vi "gRPC_Wrapper_VISA_implement_v1.1.0.vi"() -> ()   [LabVIEW 2022 SP3]
uses:
  <vilib>/Instr/_visa.llb/VISA Open Access Mode.ctl
panel:
  out "Read in sec":dbl
  out "Write in sec":dbl
  out "Round Trip Time (ms)":dbl
  out "Read time":timestamp
  out "Write time":timestamp
  in  "Refresh":bool
  in  "VISA CLOSE":bool
  in  "VISA resource name":refnum<visa-resource-name>="test_LabVIEW"
  out "Waveform Graph":dbl[](graph)
  out "Waveform Chart":dbl(graph)
  out "Gain":string
  in  "Select Command":string(combo)
  out "Active":bool
  in  "Send":bool
  in  "Type Command":string
  in  "Query":bool
  out "Command":string
  out "Dot-Notation Address":string
  out "Computer Hostname":string
  out "Resource Manufacturer Name":string
  out "Resource Manufacturer Identification":u16
  out "Version of Specification":u32
  out "Resource Lock State":u32(ring) items=["Unlocked", "Exclusive", "Shared"]
  out "Resource Name":string
  out "Read return count":u32
  out "Write return count":u32
  out "Respose From Device":string
  # "Operations"
  # "Informations"
  # "Device Signal Parameters"
  # "Graph / Chart"
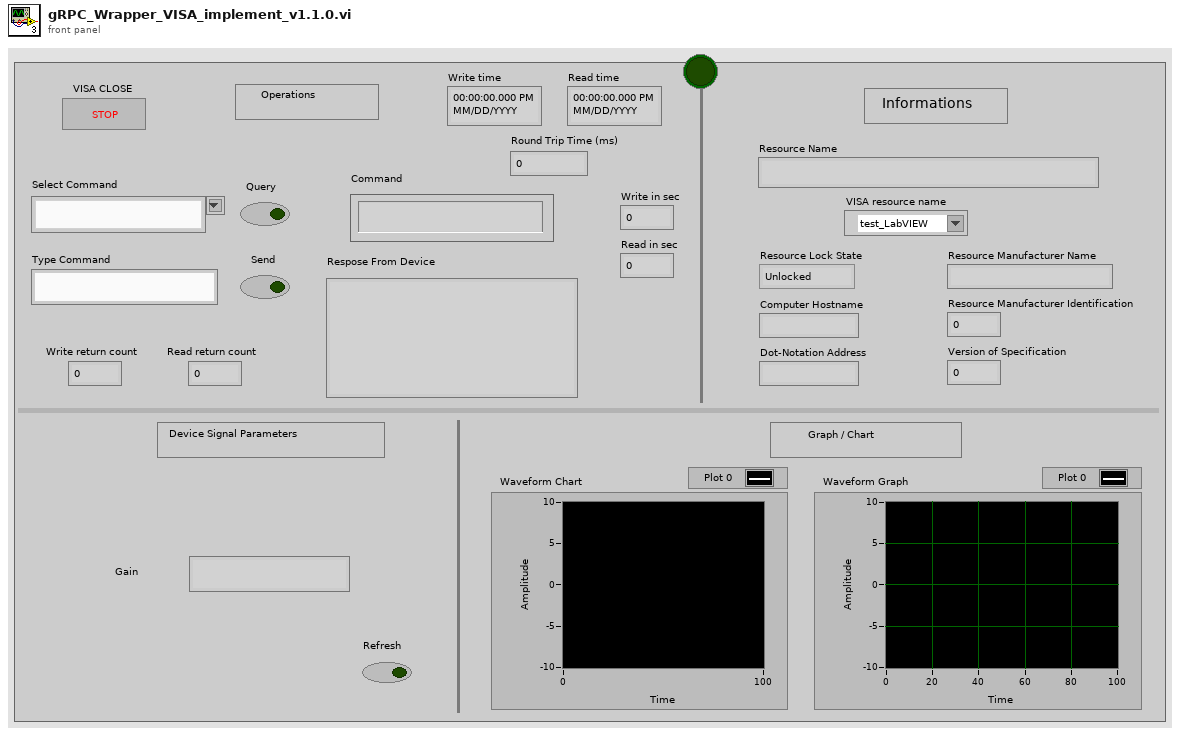
[diagram p1: front panel]
types:
  T1 = typedef "VISA Open Access Mode.ctl" = u32
  T2 = typedef "LVDateTimeRec.ctl" = cluster{"fractional second":dbl, "second":i32, "minute":i32, "hour":i32, "day of month":i32, "month":i32, "year":i32, "day of week":i32, "day of year":i32, "DST":i32}
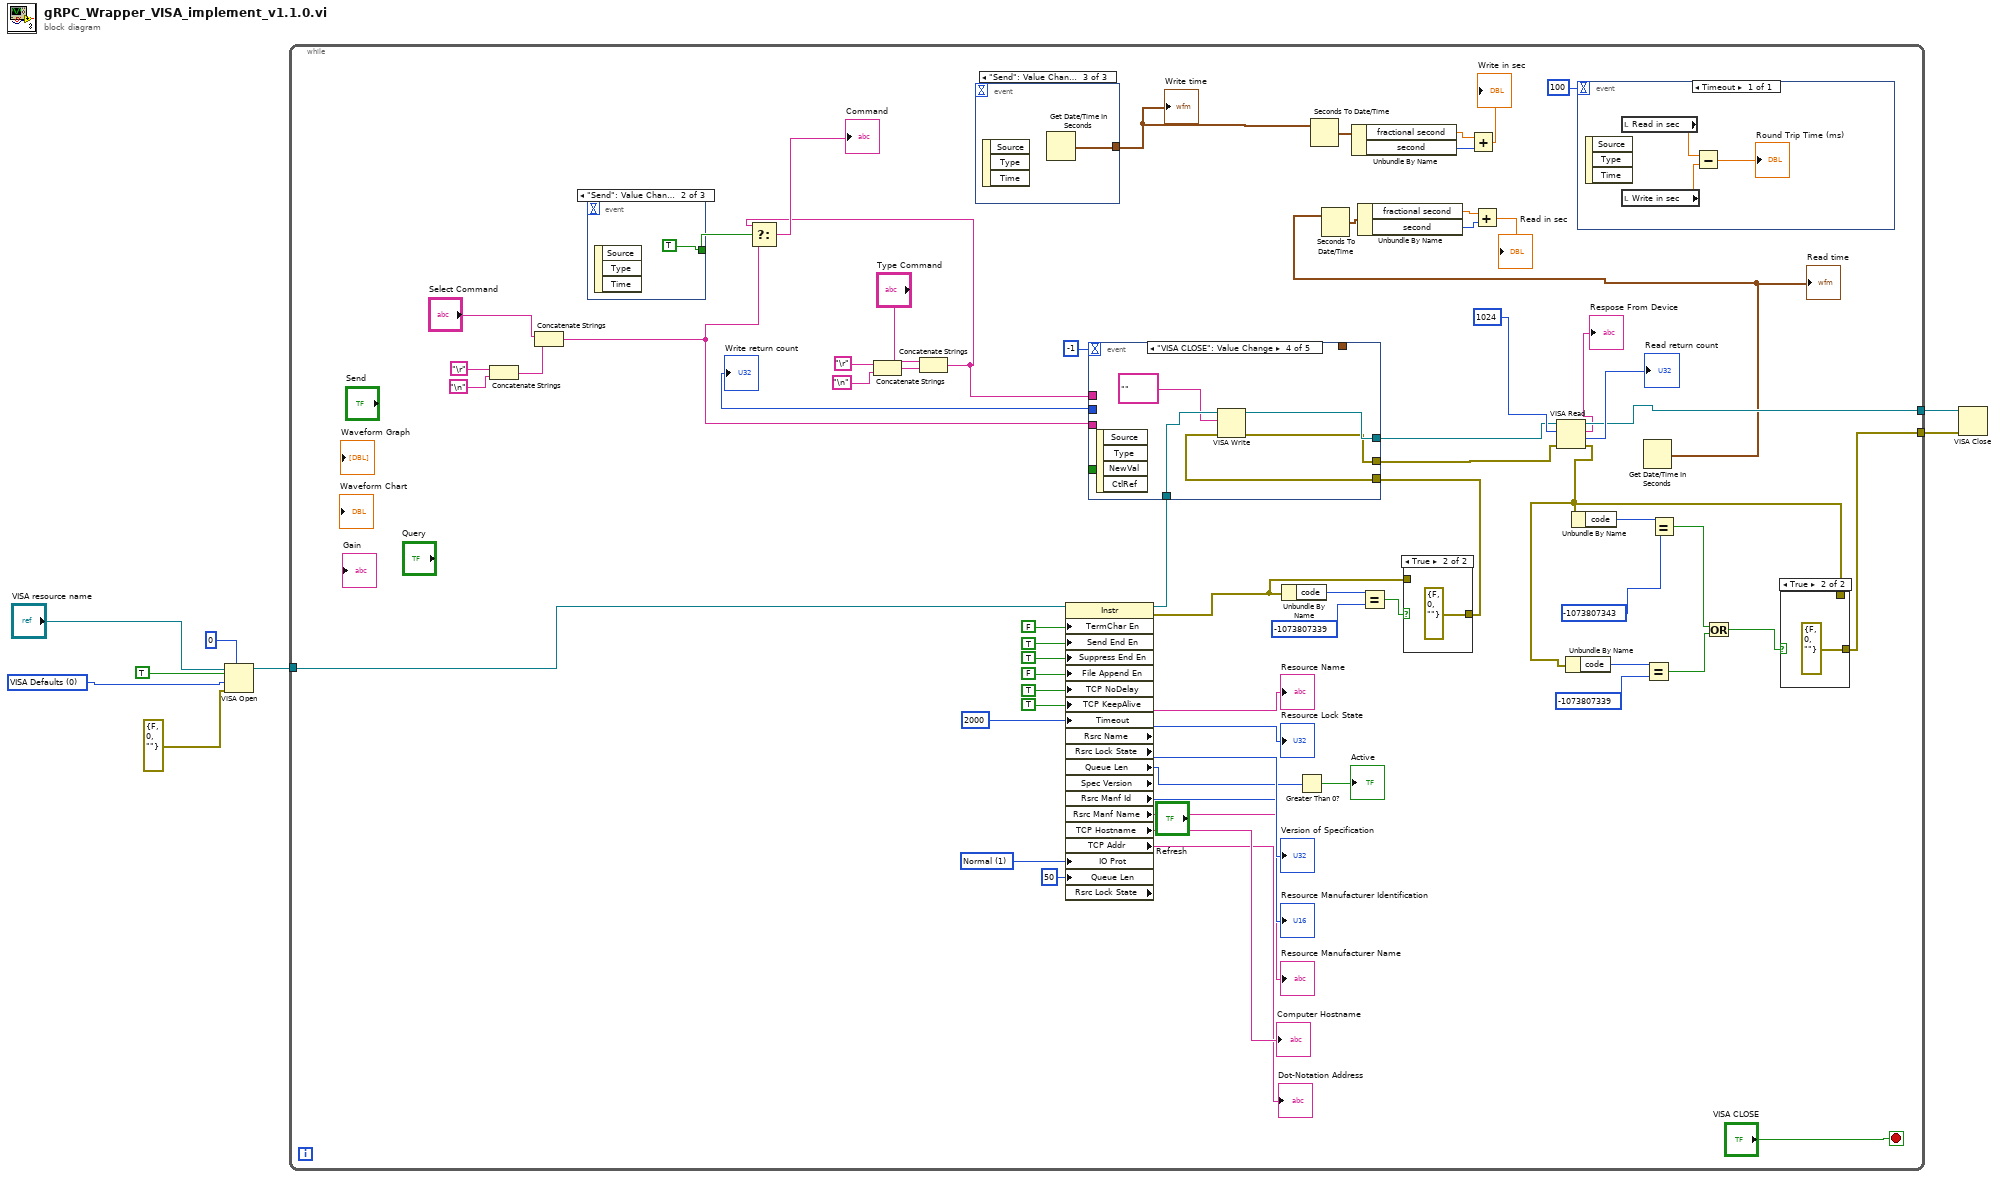
[diagram p0: block diagram]
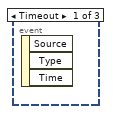
[diagram p2: hidden frame]
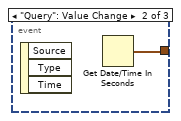
[diagram p3: hidden frame]
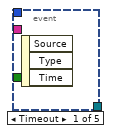
[diagram p6: hidden frame]
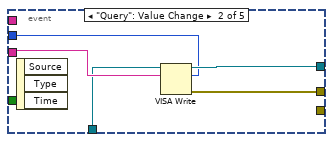
[diagram p7: hidden frame]
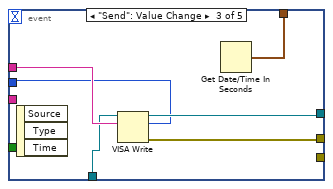
[diagram p8: hidden frame]
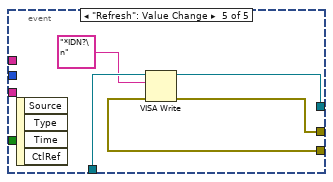
[diagram p9: hidden frame]
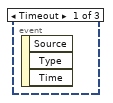
[diagram p10: hidden frame]
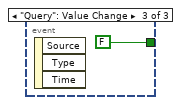
[diagram p11: hidden frame]
diagram:
  w3 = T1 0 items=["VISA Defaults"=0, "Exclusive Lock"=1, "Load Configured Settings"=4] ("Access Mode")
  n1 = VISA Open(timeout (0)=u32 0 ("VISA Open timeout (0)"), duplicate session (F)=TRUE, access mode=w3, error in (no error)=errorcluster {"status"=FALSE, "code"=0, "source"=""}, VISA resource name="VISA resource name") -> (VISA resource name=w1:refnum<visa-resource-name>)  [unwired: 1 out]
  n2 = while {
    tunnel: [w24] -> w8
    tunnel: [w23] -> w7
    tunnel: w1 -> [w22]
    stop <- "VISA CLOSE" stop-if-true
    w60 = u16 1 items=["Normal"=1, "VXI/FDC"=2, "GPIB/HS488"=3, "Serial-TCPIP-USB/488 Strings"=4, "USBTMC/Vendor-Specific"=5] ("Message Based Settings:IO Protocol")
    n3 = Concatenate Strings("\r", "\n") -> (w47:string)
    n4 = Concatenate Strings("Select Command", w47) -> (w21:string)
    n5 = event shown="[1] \"Send\": Value Change" {
      selector: _ -> [_ _ _]
      dyn-events: _ -> [_ _ _]
      timeout: _ -> [_ _ _]
      tunnel: [_ TRUE FALSE] -> w49
      event Timeout {
        n6 = event-data() -> ()  [unwired: 1 in, 3 out]
      }
      event "Send": Value Change {
        n7 = event-data() -> ()  [unwired: 1 in, 3 out]
      }
      event "Query": Value Change {
        n8 = event-data() -> ()  [unwired: 1 in, 3 out]
      }
    }
    n9 = Concatenate Strings("\r", "\n") -> (w48:string)
    n10 = Concatenate Strings("Type Command", w48) -> (w43:string)
    n11 = Select(t=w43, s=w49, f=w21) -> (s? t:f=→"Command":string)
    n12 = event shown="[2] \"Send\": Value Change" {
      selector: _ -> [_ _ _]
      dyn-events: _ -> [_ _ _]
      timeout: _ -> [_ _ _]
      tunnel: [_ w78 w79] -> w19
      event Timeout {
        n13 = event-data() -> ()  [unwired: 1 in, 3 out]
      }
      event "Query": Value Change {
        n14 = event-data() -> ()  [unwired: 1 in, 3 out]
        n15 = Get Date/Time In Seconds() -> (seconds since 1Jan1904=w78:timestamp)
      }
      event "Send": Value Change {
        n16 = event-data() -> ()  [unwired: 1 in, 3 out]
        n17 = Get Date/Time In Seconds() -> (seconds since 1Jan1904=w79:timestamp)
      }
    }
    "Write time" <- w19
    n18 = property class="Instr" props=["TermChar En", "Send End En", "Suppress End En", "File Append En", "TCP NoDelay", "TCP KeepAlive", "Timeout", "Rsrc Name", "Rsrc Lock State", "Queue Len", "Spec Version", "Rsrc Manf Id", "Rsrc Manf Name", "TCP Hostname", "TCP Addr", "IO Prot", "Queue Len", "Rsrc Lock State"](reference=w22, "TermChar En"=FALSE ("Message Based Settings:Termination Character Enable"), "Send End En"=TRUE ("Message Based Settings:Send End Enable"), "Suppress End En"=TRUE ("Message Based Settings:Suppress End Enable"), "File Append En"=FALSE ("Message Based Settings:File Append Enable"), "TCP NoDelay"=TRUE ("TCP/IP Settings:No Packet Delay"), "TCP KeepAlive"=TRUE ("TCP/IP Settings:Keep-Alive Packets"), "Timeout"=u32 2000 ("General Settings:Timeout Value"), "IO Prot"=w60, "Queue Len"=u32 50 ("General Settings:Maximum Queue Length")) -> (reference out=w42:refnum<visa-resource-name>, error out=w35:errorcluster, "Rsrc Name"=→"Resource Name":string, "Rsrc Lock State"=→"Resource Lock State":u32, "Queue Len"=w52:u32, "Spec Version"=→"Version of Specification":u32, "Rsrc Manf Id"=→"Resource Manufacturer Identification":u16, "Rsrc Manf Name"=→"Resource Manufacturer Name":string, "TCP Hostname"=→"Computer Hostname":string, "TCP Addr"=→"Dot-Notation Address":string)  [unwired: 1 in, 1 out]
    n19 = Unbundle By Name(w35) -> ("code"=w38:i32)
    n20 = Greater Than 0?(x=w52) -> (x > 0?=→"Active":bool)
    n21 = Seconds To Date/Time(time stamp (now)=w19) -> (date time rec=w18:T2)  [unwired: 1 in]
    n22 = Unbundle By Name(w18) -> ("fractional second"=w14:dbl, "second"=w13:i32)
    n23 = Equal?(x=w38, y=-1073807339) -> (x = y?=w37:bool)
    n24 = case shown="True" w37 {
      tunnel: [w80 errorcluster {"status"=FALSE, "code"=0, "source"=""} ("error constant")] -> w36
      tunnel: w35 -> [w80 _]
      frame False {
      }
      frame True {
      }
    }
    n25 = event shown="[3] \"VISA CLOSE\": Value Change" {
      selector: _ -> [_ _ _ _ _]
      dyn-events: _ -> [_ _ _ _ _]
      timeout: -1 -> [_ _ _ _ _]
      tunnel: [_ w88 w94 w100 w104] -> w26
      tunnel: [_ w87 w93 w99 w103] -> w25
      tunnel: [_ w85 w91 _ _] -> w56
      tunnel: w21 -> [_ w86 _ _ _]
      tunnel: w43 -> [_ _ w92 _ _]
      tunnel: w42 -> [_ w84 w90 w97 w105]
      tunnel: w36 -> [_ _ _ w98 w102]
      tunnel: [_ _ _ w95 _] -> _
      tunnel: [_ _ w89 _ _] -> _
      event Timeout {
        n26 = event-data() -> ()  [unwired: 1 in, 3 out]
      }
      event "Query": Value Change {
        n27 = event-data() -> ()  [unwired: 1 in, 3 out]
        n28 = VISA Write(VISA resource name=w84, write buffer=w86) -> (VISA resource name out=w88:refnum<visa-resource-name>, return count=w85:u32, error out=w87:errorcluster)  [unwired: 1 in]
      }
      event "Send": Value Change {
        n29 = event-data() -> ()  [unwired: 1 in, 3 out]
        n30 = VISA Write(VISA resource name=w90, write buffer=w92) -> (VISA resource name out=w94:refnum<visa-resource-name>, return count=w91:u32, error out=w93:errorcluster)  [unwired: 1 in]
        n31 = Get Date/Time In Seconds() -> (seconds since 1Jan1904=w89:timestamp)
      }
      event "VISA CLOSE": Value Change {
        n32 = event-data() -> ("NewVal"=w95:bool)  [unwired: 1 in, 3 out]
        n33 = VISA Write(VISA resource name=w97, write buffer="", error in (no error)=w98) -> (VISA resource name out=w100:refnum<visa-resource-name>, error out=w99:errorcluster)  [unwired: 1 out]
      }
      event "Refresh": Value Change {
        n34 = event-data() -> ()  [unwired: 1 in, 4 out]
        n35 = VISA Write(VISA resource name=w105, write buffer="*IDN?\n", error in (no error)=w102) -> (VISA resource name out=w104:refnum<visa-resource-name>, error out=w103:errorcluster)  [unwired: 1 out]
      }
    }
    "Write return count" <- w56
    n36 = Add(x=w14, y=w13) -> (x+y=→"Write in sec":dbl)
    n37 = VISA Read(VISA resource name=w26, byte count=u32 1024, error in (no error)=w25) -> (VISA resource name out=w23:refnum<visa-resource-name>, read buffer=→"Respose From Device":string, return count=→"Read return count":u32, error out=w31:errorcluster)
    n38 = Unbundle By Name(w31) -> ("code"=w32:i32)
    n39 = Unbundle By Name(w31) -> ("code"=w41:i32)
    n40 = event shown="[0] Timeout" {
      selector: _ -> [_]
      dyn-events: _ -> [_]
      timeout: 100 -> [_]
      event Timeout {
        n41 = event-data() -> ()  [unwired: 1 in, 3 out]
        n42 = local read "Read in sec"() -> (w75:dbl)
        n43 = local read "Write in sec"() -> (w76:dbl)
        n44 = Subtract(x=w75, y=w76) -> (x-y=→"Round Trip Time (ms)":dbl)
      }
    }
    n45 = Get Date/Time In Seconds() -> (seconds since 1Jan1904=w20:timestamp)
    "Read time" <- w20
    n46 = Seconds To Date/Time(time stamp (now)=w20) -> (date time rec=w17:T2)  [unwired: 1 in]
    n47 = Unbundle By Name(w17) -> ("fractional second"=w16:dbl, "second"=w15:i32)
    n48 = Add(x=w16, y=w15) -> (x+y=→"Read in sec":dbl)
    n49 = Equal?(x=w32, y=-1073807339) -> (x = y?=w28:bool)
    n50 = Equal?(x=w41, y=-1073807343) -> (x = y?=w29:bool)
    n51 = Or(x=w29, y=w28) -> (x .or. y?=w30:bool)
    n52 = case shown="True" w30 {
      tunnel: [w82 errorcluster {"status"=FALSE, "code"=0, "source"=""} ("error constant")] -> w24
      tunnel: w31 -> [w82 _]
      frame False {
      }
      frame True {
      }
    }
  }
  n53 = VISA Close(VISA resource name=w7, error in (no error)=w8) -> ()  [unwired: 1 out]
